vi "DAC Run.vi"(8 "error in":errorcluster, 11 "DAC Heater Ctrl in":refnum<class "DAC Heater Ctrl.lvclass">) -> (0 "error out":errorcluster, 3 "DAC Heater Ctrl out":refnum<class "DAC Heater Ctrl.lvclass">)   [LabVIEW 2019, in "DAC.lvlib" / "DAC Heater Ctrl.lvclass"]
uses:
  DAC Heater Ctrl.lvclass
  C:/Users/wg/Documents/LV_Projects/TestStand/App/DAC/DAC.lvclass
  DAC.lvclass/DAC.ctl
  Results/LNG Boiling Results/LNG Boiling Results.lvclass
  Results/Results Method.ctl
  DAC Heater Ctrl.lvclass/DAC Heater Ctrl.ctl
  <vilib>/DAQmx/write.llb/DAQmx Write (Analog DBL 1Chan 1Samp).vi
  <vilib>/DAQmx/miscellaneous.llb/DAQmx Fill In Error Info.vi
  DAC.lvclass
  Results/Results.lvlib
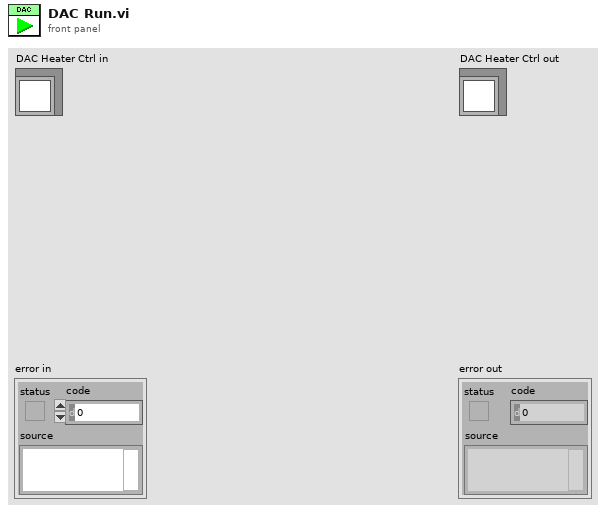
[diagram p1: front panel]
types:
  T1 = typedef "Results.lvlib/Results Method.ctl" = enum16{"Get", "Set"}
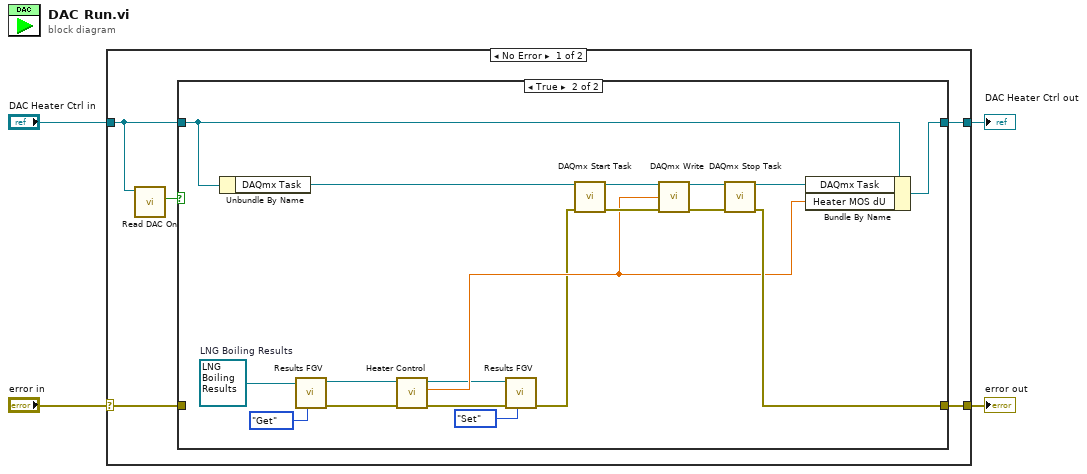
[diagram p0: block diagram]
diagram:
  n1 = case shown="No Error" "error in" {
    selector: "error in" -> [w7 w31]
    tunnel: [w6 w31] -> w2
    tunnel: [w8 w30] -> w1
    tunnel: "DAC Heater Ctrl in" -> [w5 w30]
    frame No Error {
      n2 = call "Read DAC On.vi"("DAC in"=w5) -> ("DAC On"=w9:bool)  [unwired: 8 in, 2 out]
      n3 = case shown="True" w9 {
        tunnel: w5 -> [w11 w25]
        tunnel: [w11 w20] -> w8
        tunnel: w7 -> [w10 _]
        tunnel: [w10 w19] -> w6
        frame False {
        }
        frame True {
          w24 = refnum<class "LNG Boiling Results.lvclass"> refnum  # LNG Boiling Results
          n4 = Unbundle By Name(w25) -> ("DAQmx Task"=w29:refnum<k21>)
          n5 = call-dynamic "Results FGV.vi"("Method"=Results_Method."Get", "LNG Boiling Results in"=w24) -> ("error out"=w18:errorcluster, "LNG Boiling Results out"=w17:refnum<class "LNG Boiling Results.lvclass">)  [unwired: 8 in]
          n6 = call "Heater Control.vi"("error in"=w18, "LNG Boiling Results in"=w17) -> ("error out"=w15:errorcluster, "Htr MOS Ctrl"=w16:dbl, "LNG Boiling Results out"=w12:refnum<class "LNG Boiling Results.lvclass">)  [unwired: 7 in]
          n7 = call-dynamic "Results FGV.vi"("Method"=Results_Method."Set", "error in"=w15, "LNG Boiling Results in"=w12) -> ("error out"=w14:errorcluster)  [unwired: 7 in, 1 out]
          n8 = call <vilib>:"DAQmx Start Task.vi"("task/channels in"=w29, "error in"=w14) -> ("task out"=w28:refnum<k21>, "error out"=w27:errorcluster)  [unwired: 12 in]
          n9 = call-poly <vilib>:"DAQmx Write.vi"("task/channels in"=w28, "data"=w16, "error in"=w27) -> ("task out"=w21:refnum<k21>, "error out"=w26:errorcluster)  [unwired: 10 in, 1 out]
          n10 = call <vilib>:"DAQmx Stop Task.vi"("task/channels in"=w21, "error in"=w26) -> ("task out"=w22:refnum<k21>, "error out"=w19:errorcluster)  [unwired: 12 in]
          n11 = Bundle By Name(cluster=w25, "DAQmx Task"=w22, "Heater MOS dU"=w16) -> (w20:refnum<class "DAC Heater Ctrl.lvclass">)
        }
      }
    }
    frame Error {
    }
  }
  "error out" <- w2
  "DAC Heater Ctrl out" <- w1
